vi "IGC100 Log Pressure.vi"(0 "Array":dbl[](array[numeric])) -> ()   [LabVIEW 2018]
uses:
  <vilib>/Utility/file.llb/Read Delimited Spreadsheet (string).vi
  <vilib>/Utility/file.llb/Write Delimited Spreadsheet (DBL).vi
panel:
  in  "Config File":path=path "C:/Users/Admin/Documents/IPES Control Panel/IPES Config Files/Pressure Log.conf"
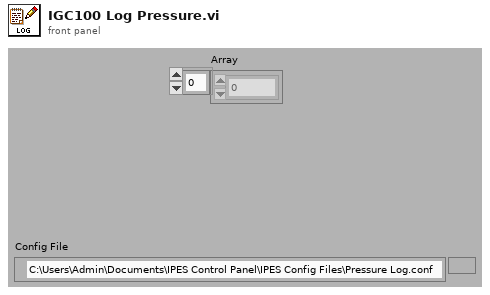
[diagram p1: front panel]
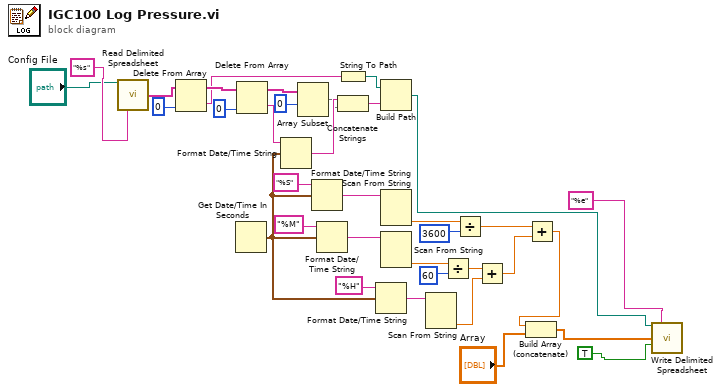
[diagram p0: block diagram]
diagram:
  n1 = call-poly <vilib>:"Read Delimited Spreadsheet.vi"("file path (dialog if empty)"="Config File", "format (%s)"="%s" ("format (%.3f)")) -> ("first row"=w4:string[])  [unwired: 8 in, 5 out]
  n2 = Delete From Array(array=w4, index=0) -> (deleted portion=w13:string, array with subset deleted=w16:string[])  [unwired: 1 in]
  n3 = Get Date/Time In Seconds() -> (seconds since 1Jan1904=w34:timestamp)
  n4 = Delete From Array(array=w16, index=0) -> (deleted portion=w10:string, array with subset deleted=w15:string[])  [unwired: 1 in]
  n5 = Format Date/Time String(time format string (%c)=w10, seconds (now)=w34) -> (date/time string=w19:string)  [unwired: 1 in]
  n6 = Array Subset(array=w15, index=0) -> (w11:string[])  [unwired: 1 in]
  n7 = Format Date/Time String(time format string (%c)="%S", seconds (now)=w34) -> (date/time string=w28:string)  [unwired: 1 in]
  n8 = Format Date/Time String(time format string (%c)="%M", seconds (now)=w34) -> (date/time string=w21:string)  [unwired: 1 in]
  n9 = String To Path(string=w13) -> (path=w12:path)
  n10 = Concatenate Strings(w19, w11) -> (w35:string)
  n11 = Format Date/Time String(time format string (%c)="%H", seconds (now)=w34) -> (date/time string=w20:string)  [unwired: 1 in]
  n12 = Build Path(base path=w12, name or relative path=w35) -> (appended path=w8:path)
  n13 = Scan From String(input string=w28) -> (output 1=w27:dbl)  [unwired: 4 in, 3 out]
  n14 = Scan From String(input string=w21) -> (output 1=w31:dbl)  [unwired: 4 in, 3 out]
  n15 = Scan From String(input string=w20) -> (output 1=w26:dbl)  [unwired: 4 in, 3 out]
  n16 = Divide(x=w31, y=60) -> (x/y=w25:dbl)
  n17 = Divide(x=w27, y=3600) -> (x/y=w23:dbl)
  n18 = Add(x=w25, y=w26) -> (x+y=w22:dbl)
  n19 = Add(x=w23, y=w22) -> (x+y=w3:dbl)
  n20 = Build Array (concatenate)(w3, "Array") -> (w1:dbl[])
  n21 = call-poly <vilib>:"Write Delimited Spreadsheet.vi"("file path (dialog if empty)"=w8, "format (%.3f)"="%e", "1D data"=w1, "append to file? (new file:F)"=TRUE) -> ()  [unwired: 10 in, 2 out]
